vi "Combine Channels.vi"(8 "error in (no error)":errorcluster, 10 "Channels (CH1+CH2) Combinations":u16(ring)=1 items=["Track", "Series", "Parallel", "Combination Off"], 11 "VISA resource name":refnum<visa-resource-name>) -> (0 "error out":errorcluster, 3 "VISA resource name out":refnum<visa-resource-name>)   [LabVIEW 2018, in "Keithley KE22xx Series.lvlib"]
doc: "Set the instrument Channel 1 and Channel 2 in various Combination States.\n\n1. Track State \n2. Series State\n3. Parallel State\n4. Combination Off."
uses:
  Keithley KE22xx Series.lvlib
panel:
  # "© 2012 Keithley Instruments, Inc. ALL RIGHTS RESERVED"
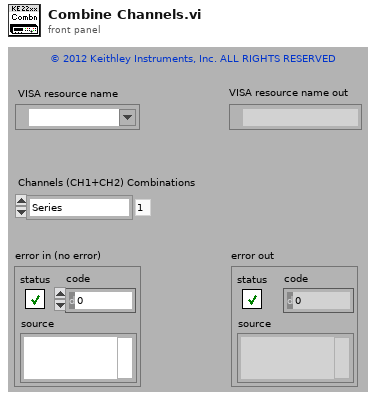
[diagram p1: front panel]
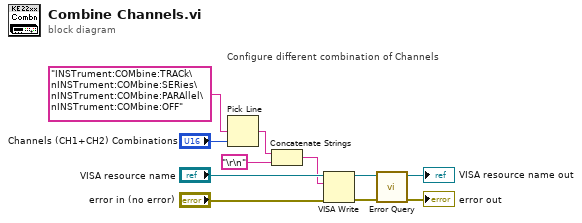
[diagram p0: block diagram]
diagram:
  # "Configure different combination of Channels"
  n1 = Pick Line(multi-line string="INSTrument:COMbine:TRACk\nINSTrument:COMbine:SERies\nINSTrument:COMbine:PARAllel\nINSTrument:COMbine:OFF", line index="Channels (CH1+CH2) Combinations") -> (output string=w7:string)  [unwired: 1 out]
  n2 = Concatenate Strings(w7, "\r\n") -> (w6:string)
  n3 = VISA Write(VISA resource name="VISA resource name", write buffer=w6, error in (no error)="error in (no error)") -> (VISA resource name out=w4:refnum<visa-resource-name>, error out=w3:errorcluster)  [unwired: 1 out]
  n4 = call "Error Query.vi"("error in (no error)"=w3, "VISA resource name"=w4) -> ("error out"=→"error out":errorcluster, "VISA resource name out"=→"VISA resource name out":refnum<visa-resource-name>)  [unwired: 6 in, 2 out]
